vi "Read Mission Controller Settings Message.vi"(8 "error in (no error)":errorcluster, 11 "Set Mission Controller Settings Message in":refnum<class "Set Mission Controller Settings Message.lvclass">) -> (0 "error out":errorcluster, 2 "Mission Controller Settings":T1, 3 "Set Mission Controller Settings Message out":refnum<class "Set Mission Controller Settings Message.lvclass">)   [LabVIEW 2015, in "RDS Child Messages.lvlib" / "Set Mission Controller Settings Message.lvclass"]
uses:
  Set Mission Controller Settings Message.lvclass
  RDS Mission Controller Actor/Mission Controller Settings.ctl
  Set Mission Controller Settings Message.lvclass/Set Mission Controller Settings Message.ctl
  RDS Mission Controller Actor/RDS Mission Controller Actor.lvlib
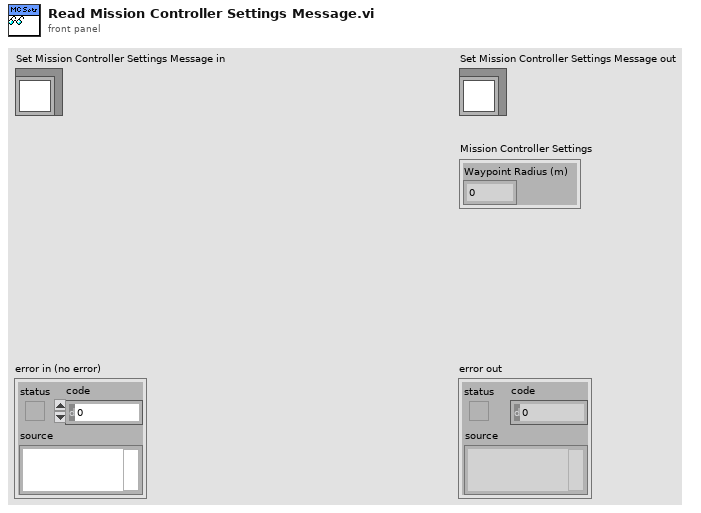
[diagram p1: front panel]
types:
  T1 = typedef "RDS Mission Controller Actor.lvlib/Mission Controller Settings.ctl" = cluster{"Waypoint Radius (m)":dbl}
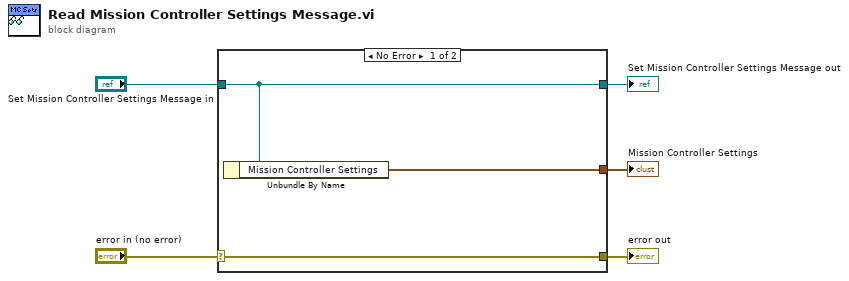
[diagram p0: block diagram]
diagram:
  n1 = case shown="No Error" "error in (no error)" {
    selector: "error in (no error)" -> [w8 w9]
    tunnel: [w8 w9] -> w4
    tunnel: [w7 w10] -> w2
    tunnel: "Set Mission Controller Settings Message in" -> [w7 w10]
    tunnel: [w6 _] -> w1
    frame No Error {
      n2 = Unbundle By Name(w7) -> ("Mission Controller Settings"=w6:T1)
    }
    frame Error {
    }
  }
  "error out" <- w4
  "Set Mission Controller Settings Message out" <- w2
  "Mission Controller Settings" <- w1
